vi "UI Send Action.vi"(8 "error in (no error)":errorcluster, 9 "Action Data":variant, 10 "UI Actions":T2, 11 "Controller in":refnum<class "Controller.lvclass">) -> (0 "error out":errorcluster, 3 "Controller out":refnum<class "Controller.lvclass">)   [LabVIEW 2020, in "Controller.lvlib" / "Controller.lvclass"]
uses:
  Controller.lvclass
  Main_UI/Main_UI/UI Actions.ctl
  Main_UI/PCRamCellNo.ctl
  Controller.lvclass/Controller.ctl
  DataPool/CycleState.ctl
  Main_UI/Main_UI Messages/Update Cycle States Msg/Update Cycle States Msg.lvclass/Update Cycle States Msg.ctl
  <vilib>/ActorFramework/Message Enqueuer/Message Enqueuer.lvclass/Message Enqueuer.ctl
  Actor_NI6008/Actor_NI6008 Messages/NI6008 DUT Switch Msg/NI6008 DUT Switch Msg.lvclass/NI6008 DUT Switch Msg.ctl
  Actor_log/Actor_log Messages/Write Event to Log Msg/Write Event to Log Msg.lvclass/Write Event to Log Msg.ctl
  <vilib>/ActorFramework/Message Enqueuer/Enqueue.vi
  Main_UI/Main_UI Messages/Update Cycle States Msg/Update Cycle States Msg.lvclass
  C:/Program Files/National Instruments/LabVIEW 2020/vi.lib/ActorFramework/Message/Message.lvclass
  Actor_NI6008/Actor_NI6008 Messages/NI6008 DUT Switch Msg/NI6008 DUT Switch Msg.lvclass
  Actor_log/Actor_log Messages/Write Event to Log Msg/Write Event to Log Msg.lvclass
  <vilib>/ActorFramework/Message Priority Queue/Priority Enqueue.vi
  Main_UI/Main_UI/Main_UI.lvclass
panel:
  out "PCMcell":T1=enum."Cell 1"
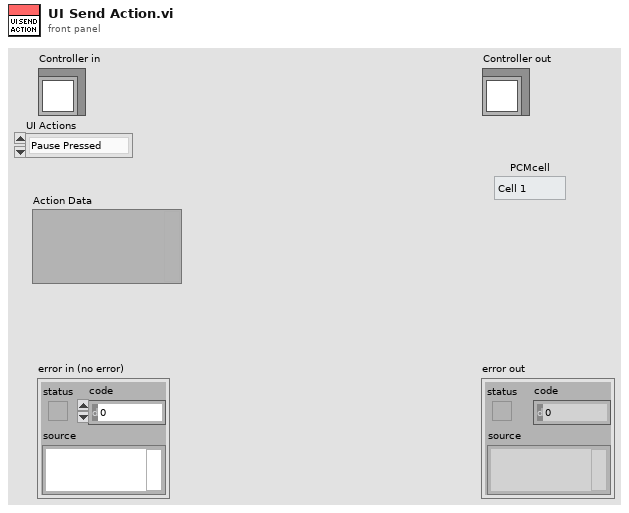
[diagram p1: front panel]
types:
  T1 = typedef "Main_UI.lvlib/Main_UI.lvclass/PCRamCellNo.ctl" = enum16{"Open All", "Cell 1", "Cell 2", "Cell 3", "Cell 4"}
  T2 = typedef "Main_UI.lvlib/Main_UI.lvclass/UI Actions.ctl" = enum16{"Pause Pressed", "Write Pressed", "RV Send Pressed", "Save Data Pressed", "Self Test Pressed", "PCRam Cell No. Changed"}
  T3 = typedef "DataPool.lvlib/CycleState.ctl" = enum16{"Idle", "Running", "Paused", "Inactive"}
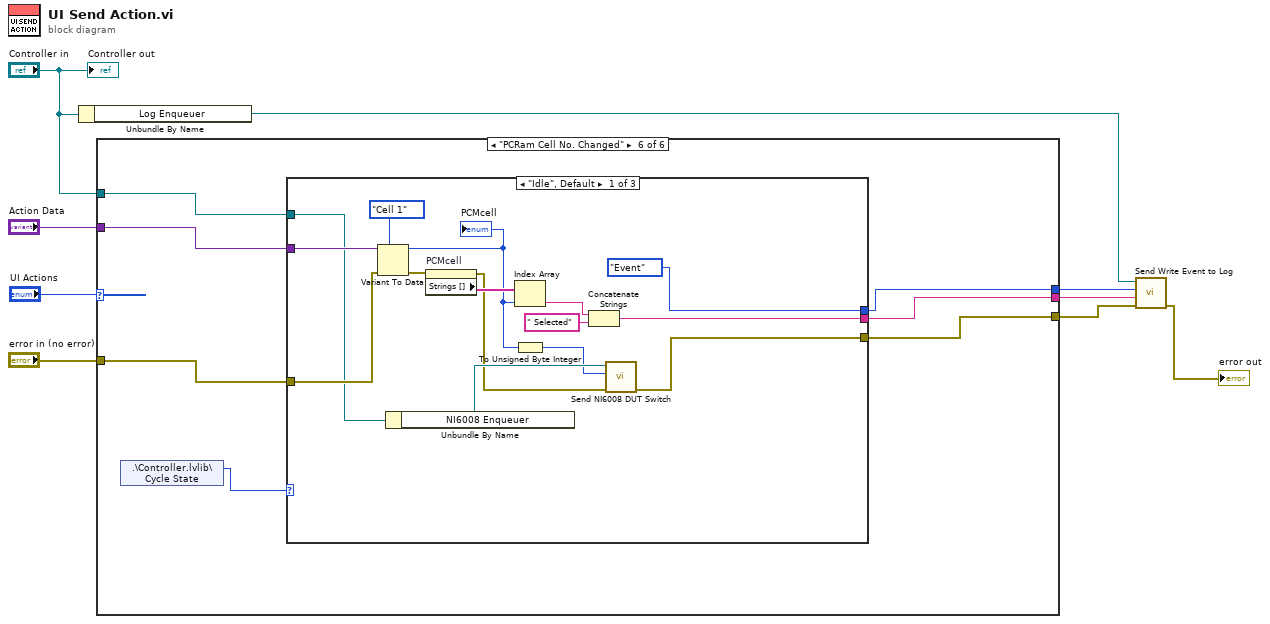
[diagram p0: block diagram]
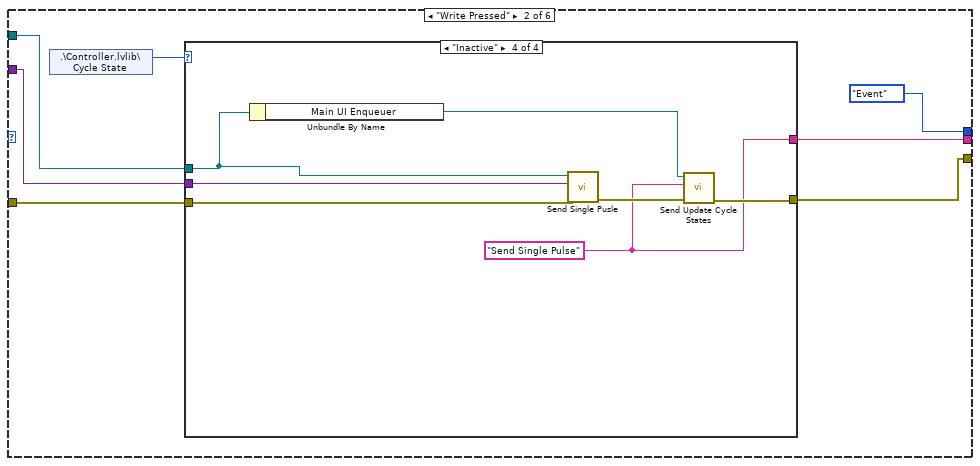
[diagram p3: hidden frame]
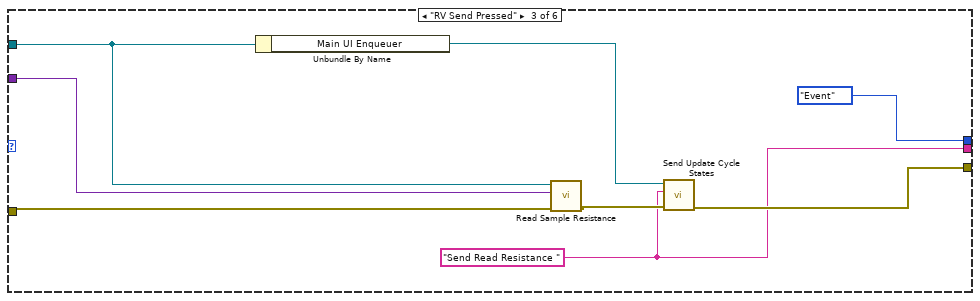
[diagram p7: hidden frame]
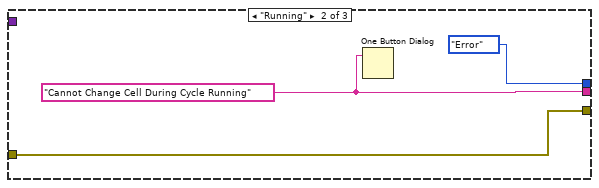
[diagram p10: hidden frame]
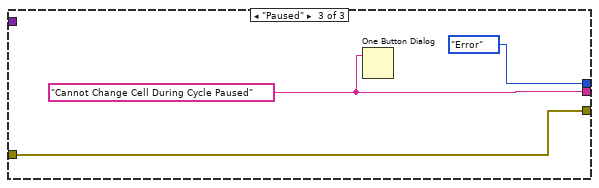
[diagram p11: hidden frame]
diagram:
  n1 = Unbundle By Name("Controller in") -> ("Log Enqueuer"=w7:refnum<class "Message Enqueuer.lvclass">)
  n2 = case shown="\"PCRam Cell No. Changed\"" "UI Actions" {
    tunnel: "Action Data" -> [_ w17 w30 _ _ w42]
    tunnel: [_ w12 w26 _ _ w41] -> w5
    tunnel: [_ enum16{"Event", "Error"}."Event" ("Enum") enum16{"Event", "Error"}."Event" ("Enum") _ _ w40] -> w6
    tunnel: [w10 w14 w28 w34 w35 w37] -> w4
    tunnel: "error in (no error)" -> [w10 w16 w33 w34 w35 w39]
    tunnel: "Controller in" -> [_ w15 w31 _ _ w38]
    frame "Pause Pressed", Default {
    }
    frame "Write Pressed" {
      n3 = shared-variable ".\\Controller.lvlib\\Cycle State"() -> (w13:T3)  [unwired: 1 in, 1 out]
      n4 = case shown="\"Inactive\"" w13 {
        tunnel: w17 -> [_ _ _ w25]
        tunnel: w16 -> [_ w18 _ w24]
        tunnel: w15 -> [_ _ _ w23]
        tunnel: [_ w18 _ w20] -> w14
        tunnel: [_ _ _ w19] -> w12
        frame "Idle", Default {
        }
        frame "Running" {
        }
        frame "Paused" {
        }
        frame "Inactive" {
          w19 = "Send Single Pulse" ("Cycle State Message")
          n5 = Unbundle By Name(w23) -> ("Main UI Enqueuer"=w22:refnum<class "Message Enqueuer.lvclass">)
          n6 = call "Send Single Pusle.vi"("error in (no error)"=w24, "Action Data"=w25, "Controller in"=w23) -> ("error out"=w21:errorcluster)  [unwired: 8 in]
          n7 = call "Send Update Cycle States.vi"("error in (no error)"=w21, "Cycle State Message"=w19, "Message Enqueuer"=w22) -> ("error out"=w20:errorcluster)  [unwired: 7 in, 1 out]
        }
      }
    }
    frame "RV Send Pressed" {
      w26 = "Send Read Resistance " ("Cycle State Message")
      n8 = Unbundle By Name(w31) -> ("Main UI Enqueuer"=w29:refnum<class "Message Enqueuer.lvclass">)
      n9 = call-dynamic "Read Sample Resistance.vi"("error in (no error)"=w33, "Action Data"=w30, "Controller in"=w31) -> ("error out"=w32:errorcluster)  [unwired: 7 in, 1 out]
      n10 = call "Send Update Cycle States.vi"("error in (no error)"=w32, "Cycle State Message"=w26, "Message Enqueuer"=w29) -> ("error out"=w28:errorcluster)  [unwired: 7 in, 1 out]
    }
    frame "Save Data Pressed" {
    }
    frame "Self Test Pressed" {
    }
    frame "PCRam Cell No. Changed" {
      n11 = shared-variable ".\\Controller.lvlib\\Cycle State"() -> (w36:T3)  [unwired: 1 in, 1 out]
      n12 = case shown="\"Idle\", Default" w36 {
        tunnel: w42 -> [w56 _ _]
        tunnel: [w51 w58 w61] -> w41
        tunnel: [enum16{"Event", "Error"}."Event" ("Enum") enum16{"Event", "Error"}."Error" ("Enum") enum16{"Event", "Error"}."Error" ("Enum")] -> w40
        tunnel: w39 -> [w49 w60 w63]
        tunnel: w38 -> [w47 _ _]
        tunnel: [w45 w60 w63] -> w37
        frame "Idle", Default {
          n13 = Variant To Data(error in=w49, type=PCRamCellNo."Cell 1" ("PCRam Cell No."), Variant=w56) -> (data=w44:T1, error out=w55:errorcluster)
          "PCMcell" <- w44
          n14 = Unbundle By Name(w47) -> ("NI6008 Enqueuer"=w48:refnum<class "Message Enqueuer.lvclass">)
          n15 = property on="PCMcell" class="Enum (strict)"(error in=w55) -> (error out=w46:errorcluster, "Strings []"=w54:string[])  [unwired: 1 in, 1 out]
          n16 = Index Array(array=w54, index=w44) -> (element=w53:string)
          n17 = To Unsigned Byte Integer(number=w44) -> (unsigned 8bit integer=w43:u8)
          n18 = Concatenate Strings(w53, " Selected" ("string")) -> (w51:string)
          n19 = call "Send NI6008 DUT Switch.vi"("error in (no error)"=w46, "DUT No."=w43, "Message Enqueuer"=w48) -> ("error out"=w45:errorcluster)  [unwired: 7 in, 1 out]
        }
        frame "Running" {
          w58 = "Cannot Change Cell During Cycle Running"
          n20 = One Button Dialog(message=w58) -> ()  [unwired: 1 in, 1 out]
        }
        frame "Paused" {
          w61 = "Cannot Change Cell During Cycle Paused"
          n21 = One Button Dialog(message=w61) -> ()  [unwired: 1 in, 1 out]
        }
      }
    }
  }
  n22 = call "Send Write Event to Log.vi"("error in (no error)"=w4, "Log Event Details"=w5, "Enum"=w6, "Message Enqueuer"=w7) -> ("error out"=→"error out":errorcluster)  [unwired: 6 in, 1 out]
  "Controller out" <- "Controller in"
